vi "Set Encoder Counts.vi"(5 "Encoder Count at Zero":dbl, 7 "PPR":dbl, 11 "Angle(0-1) in":T1 {"Angle" scale format="%.3f"; "Velocity" scale=-1.0..1.0 scale format="%.1f"}) -> (3 "Encder Count Set":dbl)   [LabVIEW 2020, in "SwerveDrive_ACT.lvlib"]
uses:
  SwerveDrive_ACT.lvlib
  Shared Code/TypeDefs/Cluster_Module Velocity-Direction-Rotations.ctl
  Shared Code/TypeDefs/Level_Velocity plus-minus 1.ctl
  Shared Code/TypeDefs/Dial_Compase heading unit circle CCW positive.ctl
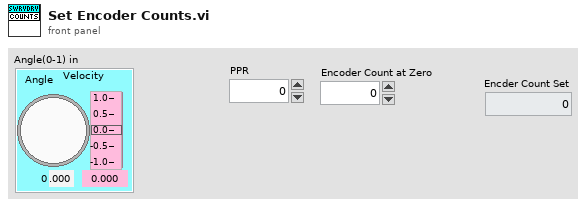
[diagram p1: front panel]
types:
  T1 = typedef "Cluster_Module Velocity-Direction-Rotations.ctl" = cluster{"Velocity":T2, "Angle":T3, "Rotations Count":dbl}
  T2 = typedef "Level_Velocity plus-minus 1.ctl" = dbl
  T3 = typedef "Dial_Compase heading unit circle CCW positive.ctl" = dbl
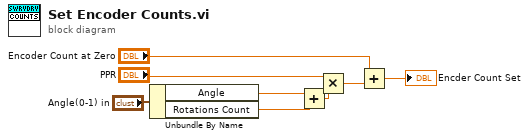
[diagram p0: block diagram]
diagram:
  n1 = Unbundle By Name("Angle(0-1) in") -> ("Angle"=w3:T3, "Rotations Count"=w2:dbl)
  n2 = Add(x=w3, y=w2) -> (x+y=w4:T3)
  n3 = Multiply(x="PPR", y=w4) -> (x*y=w6:T3)
  n4 = Add(x="Encoder Count at Zero", y=w6) -> (x+y=→"Encder Count Set":T3)
